vi "Write FWCS_ACS_Iterator.lvclass.vi"(8 "error in (no error)":errorcluster, 10 "FWCS_ACS_Iterator.lvclass":refnum<class "FWCS_ACS_Iterator.lvclass">, 11 "SPARC4_GEI in":refnum<class "SPARC4_GEI.lvclass">) -> (0 "error out":errorcluster, 3 "SPARC4_GEI out":refnum<class "SPARC4_GEI.lvclass">)   [LabVIEW 2018, in "SPARC4_GEI.lvclass"]
uses:
  SPARC4_GEI.lvclass
  FWCS_ACS_Iterator/FWCS_ACS_Iterator.lvclass
  SPARC4_GEI.lvclass/SPARC4_GEI.ctl
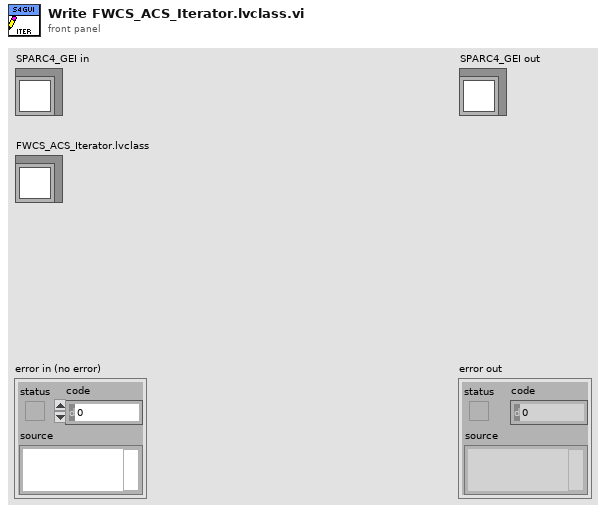
[diagram p1: front panel]
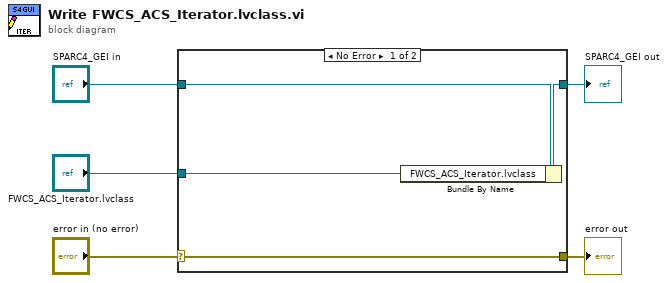
[diagram p0: block diagram]
diagram:
  n1 = case shown="No Error" "error in (no error)" {
    selector: "error in (no error)" -> [w9 w10]
    tunnel: [w9 w10] -> w4
    tunnel: [w7 w11] -> w2
    tunnel: "SPARC4_GEI in" -> [w8 w11]
    tunnel: "FWCS_ACS_Iterator.lvclass" -> [w6 _]
    frame No Error {
      n2 = Bundle By Name(cluster=w8, "FWCS_ACS_Iterator.lvclass"=w6) -> (w7:refnum<class "SPARC4_GEI.lvclass">)
    }
    frame Error {
    }
  }
  "error out" <- w4
  "SPARC4_GEI out" <- w2
